vi "SetKeyValue_Int32.vi"(6 "value":i32, 9 "key":string, 10 "key value pairs":T1[](array[typedef])) -> (2 "key value pairs out":T1[](array[typedef]))   [LabVIEW 2017, in "PropertyHelpers.lvlib"]
doc: "Writes the 32-bit signed integer value of a particular property/key in an array of key-value pairs. These VIs are useful for defining properties that the device sends to NI InsightCM Server in the form of key-value pairs within NI InsightCM message bus messages."
uses:
  <vilib>/addons/InsightCM/Utilities/PropertyHelpers/PropertyHelpers.lvlib
  <vilib>/addons/InsightCM/MessageBus/Base/controls/KeyValuePair.ctl
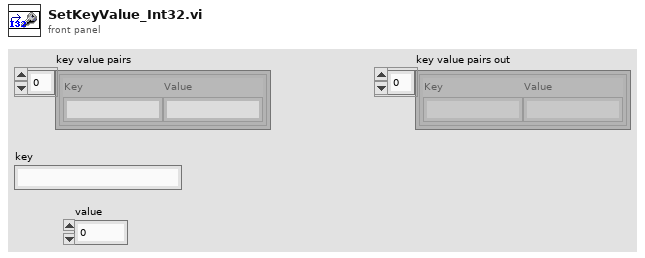
[diagram p1: front panel]
types:
  T1 = typedef "KeyValuePair.ctl" = cluster{"Key":string, "Value":string}
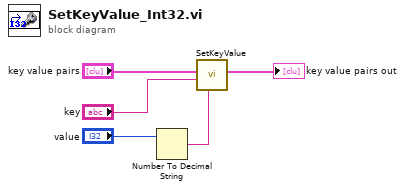
[diagram p0: block diagram]
diagram:
  n1 = Number To Decimal String(number="value") -> (decimal integer string=w1:string)  [unwired: 1 in]
  n2 = call <vilib>:"SetKeyValue.vi"("value"=w1, "key"="key", "key value pairs"="key value pairs") -> ("key value pairs out"=→"key value pairs out":T1[])  [unwired: 8 in]
